vi "myRIO_BRig_FPGA_v3,41.vi"() -> ()   [LabVIEW 2014]
uses:
  <vilib>/rvi/FXPMathLib/FxpDiv/subVIs/nifxpmath_Div_SimConfig.ctl
  <vilib>/rvi/FXPMathLib/FxpSinAndCos/subVIs/nifxpmath_SinAndCos_SimConfig.ctl
  <vilib>/rvi/FXPMathLib/FxpDiv/simVIs/DllFxpDivTemp_sub.vi
  <vilib>/rvi/FXPMathLib/FxpSinAndCos/simVIs/DllFxpSinAndCosTemp_sub.vi
  <vilib>/rvi/Emulation/niFpgaGetClockAttributes.vi
  <vilib>/rvi/Emulation/niFpgaSctlEmulationGetInTimedLoop.vi
  <vilib>/rvi/Emulation/niFpgaEmulationReportErrorSimple.vi
  <vilib>/rvi/eio/common/nirviEmuTemplateMethod_errors.vi
  <vilib>/rvi/Emulation/niFpgaCriticalErrorInLSC.vi
  <vilib>/rvi/FXPMathLib/FxpDiv/XNode/nifxpmath_Div.xnode
  <vilib>/rvi/FXPMathLib/FxpMul/XNode/nifxpmath_Multiplier.xnode
  <vilib>/rvi/FXPMathLib/FxpSinAndCos/XNode/nifxpmath_SinAndCos.xnode
  <vilib>/rvi/FXPMathLib/FxpSub/XNode/nifxpmath_Sub.xnode
  <vilib>/eio/EIONode/EIONode.xnode
  <vilib>/rvi/FXPMathLib/sim/FxpSim.dll
panel:
  in  "laser_Nshutter":u32=100
  in  "AnaOut_0":u16
  in  "laser_Nvalley":u32=100
  in  "laser_Npeak":u32=100
  in  "laserledMTrig":bool
  in  "laser_selWro_Ntotal":u32=100
  in  "laser_selWro_NDelay":u32
  in  "laser_selRew_Ntotal":u32=100
  in  "laser_selRew_Ndelay":u32
  in  "laserResponse_reward_LED":bool
  in  "laserResponse_wrong_LED":bool
  out "SelectWrong":bool
  out "SelectReward":bool
  in  "laserResponse_wrong":bool
  in  "laserResponse_reward":bool
  in  "Left(F)_or_Right(T)":bool
  in  "ignoreWrong":bool
  in  "SelectionState":bool
  in  "laserMTrig":bool
  in  "FPGA_Stop":bool
  in  "audioTrigger_L":bool
  in  "audioTrigger_R":bool
  in  "audioFreq_L_Hz":u16=1000 min=1000 max=14000 step=1000
  in  "audioAmp_L":u16=1 min=1 max=32767 step=1
  in  "audioFreq_R_Hz":u16=1000 min=1000 max=14000 step=1000
  in  "audioAmp_R":u16=1 min=1 max=32767 step=1
  in  "A3_SL":bool
  in  "A1_SR":bool
  in  "Counts_Reset":bool
  out "A4_LickR":u32
  out "A2_LickL":u32
  in  "A6_Act":bool
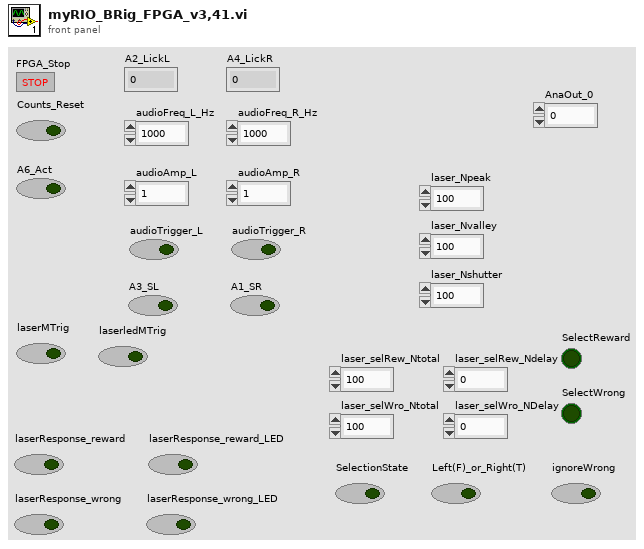
[diagram p1: front panel]
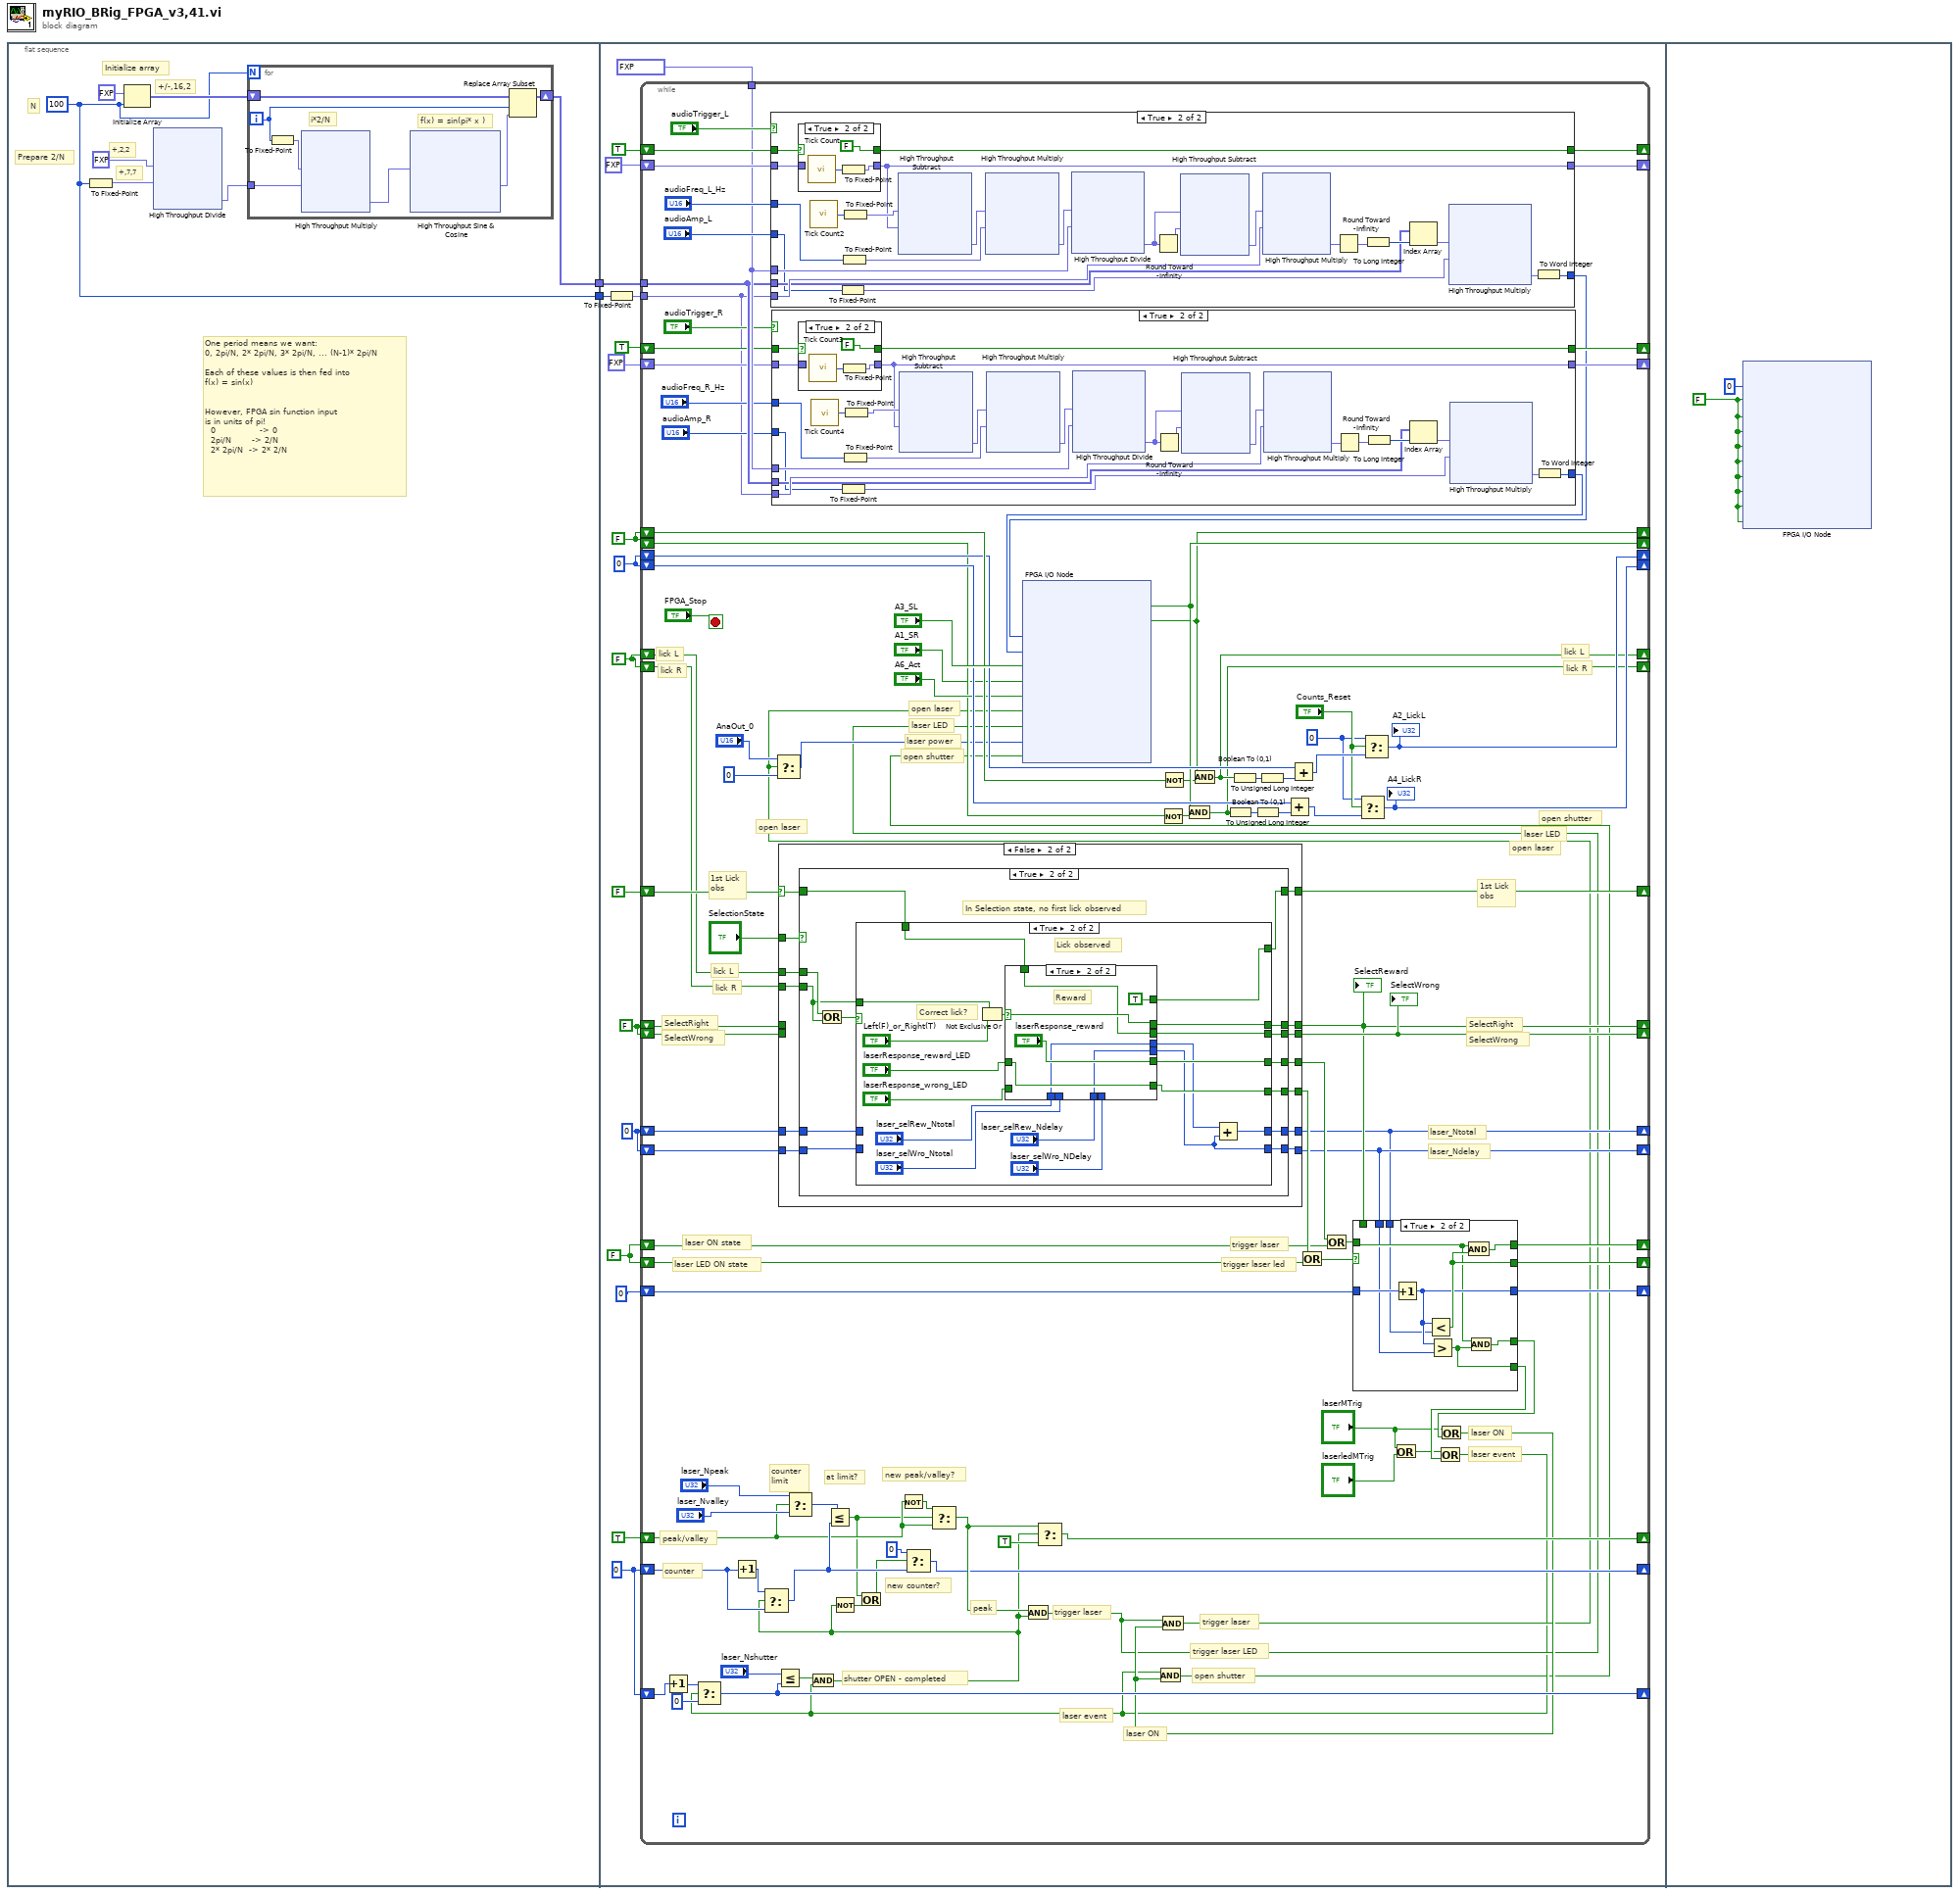
[diagram p0: block diagram]
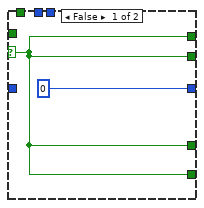
[diagram p2: hidden frame]
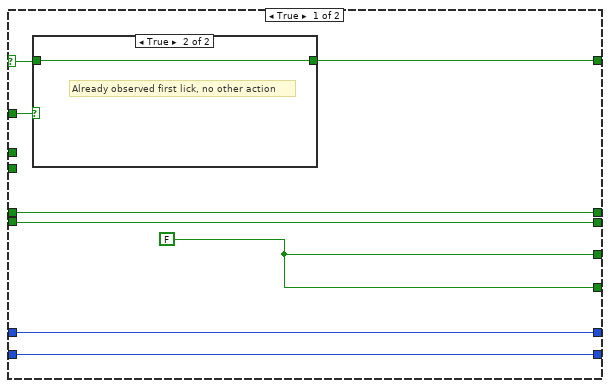
[diagram p3: hidden frame]
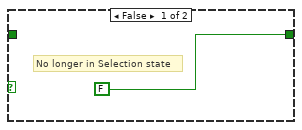
[diagram p4: hidden frame]
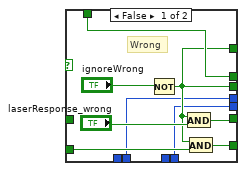
[diagram p7: hidden frame]
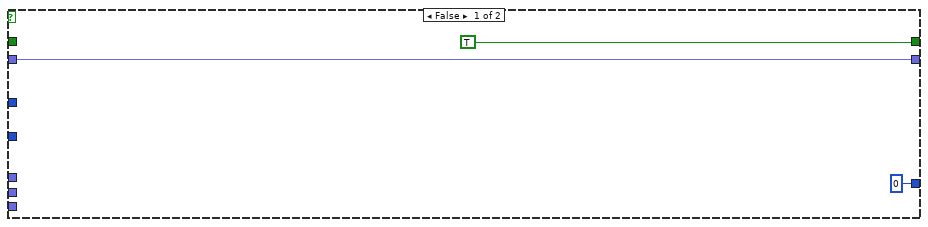
[diagram p8: hidden frame]
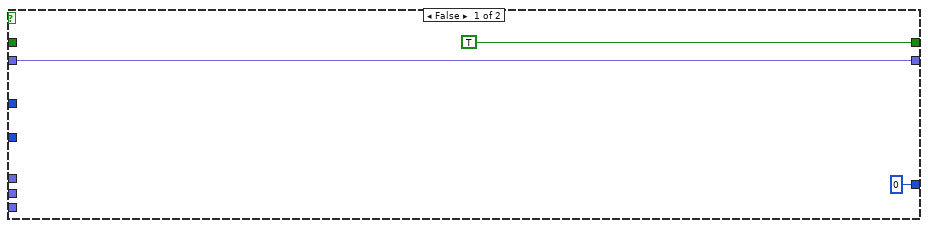
[diagram p10: hidden frame]
diagram:
  n1 = flat-sequence {
    tunnel: [w4] -> w2
    tunnel: [w3] -> w1
    tunnel: w2 -> [w86]
    tunnel: w1 -> [w88]
    frame #0 {
      w3 = 100 ("dimension size")
      # "N"
      # "+,7,7"
      # "+,2,2"
      # "+/-,16,2"
      # "Prepare 2/N"
      # "One period means we want:\n0, 2pi/N, 2* 2pi/N, 3* 2pi/N, ... (N-1)* 2pi/N\n\nEach of these values is then fed into\nf(x) = sin(x)\n\n\nHowever, FPGA sin function input\nis in units of pi!\n  0               -> 0\n  2pi/N       -> 2/N\n  2* 2pi/N  -> 2* 2/N"
      # "Initialize array"
      n2 = To Fixed-Point(number=w3) -> (fixed-point=w6:fxp<+,7,7>)  [unwired: 1 in]
      n3 = Initialize Array(fxp<+/-,16,2> 0.0 ("element"), w3) -> (w9:fxp<+/-,16,2>[])
      n4 = xnode "High Throughput Divide"("x"=fxp<+,2,2> 2.0, "y"=w6) -> ("x/y"=w5:fxp<+,27,0>)
      n5 = for {
        N: w3 -> [_]
        shift-right: [w42] -> w4
        shift-left: w9 -> [w43]
        tunnel: w5 -> [w38]
        i -> [w41]
        # "f(x) = sin(pi* x )"
        # "i*2/N"
        n6 = To Fixed-Point(number=w41) -> (fixed-point=w39:fxp<+,7,7>)  [unwired: 1 in]
        n7 = xnode ("High Throughput Multiply")("x"=w39, "y"=w38) -> ("x*y"=w37:fxp<+,34,7>)
        n8 = xnode "High Throughput Sine & Cosine"("x (pi)"=w37) -> ("sin(x)"=w40:fxp<+/-,16,2>)  [unwired: 1 out]
        n9 = Replace Array Subset(array=w43, new element=w40, index=w41) -> (w42:fxp<+/-,16,2>[])
      }
    }
    frame #1 {
      w74 = u32 0
      w76 = u32 0
      w78 = FALSE
      w77 = FALSE
      w81 = FALSE
      w82 = FALSE
      w83 = u32 0
      n10 = To Fixed-Point(number=w88) -> (fixed-point=w87:fxp<+,7,7>)  [unwired: 1 in]
      n11 = while {
        shift-right: [w187] -> _
        shift-left: TRUE -> [w191]
        shift-right: [w186] -> _
        shift-left: fxp<+,32,32> 0.0 -> [w190]
        tunnel: fxp<+,17,26> 40000000.0 -> [w185]
        tunnel: w87 -> [w178]
        tunnel: w86 -> [w184]
        shift-right: [w177] -> _
        shift-left: TRUE -> [w183]
        shift-right: [w176] -> _
        shift-left: fxp<+,32,32> 0.0 -> [w182]
        shift-right: [w154] -> _
        shift-left: w83 -> [w166]
        shift-right: [w157] -> _
        shift-left: w83 -> [w170]
        shift-right: [w158] -> _
        shift-left: w82 -> [w161]
        shift-right: [w155] -> _
        shift-left: w82 -> [w167]
        shift-right: [w152] -> _
        shift-left: FALSE -> [w151]
        shift-right: [w150] -> _
        shift-left: w81 -> [w148]
        shift-right: [w149] -> _
        shift-left: w81 -> [w147]
        shift-right: [w137] -> _
        shift-left: w77 -> [w139]
        shift-right: [w145] -> _
        shift-left: u32 0 -> [w146]
        shift-right: [w131] -> _
        shift-left: w78 -> [w143]
        shift-right: [w144] -> _
        shift-left: w78 -> [w142]
        shift-right: [w138] -> _
        shift-left: w77 -> [w135]
        shift-right: [w127] -> _
        shift-left: w76 -> [w130]
        shift-right: [w128] -> _
        shift-left: w76 -> [w129]
        shift-right: [w111] -> _
        shift-left: w74 -> [w121]
        shift-right: [w112] -> _
        shift-left: TRUE -> [w115]
        shift-right: [w100] -> _
        shift-left: w74 -> [w104]
        stop <- "FPGA_Stop" stop-if-true
        w163 = u32 0
        # "open shutter"
        # "laser LED"
        # "open laser"
        # "open laser"
        # "trigger laser LED"
        # "trigger laser"
        # "open shutter"
        # "laser ON"
        # "laser power"
        # "open laser"
        # "laser LED"
        # "open shutter"
        # "shutter OPEN - completed"
        # "trigger laser"
        # "peak"
        # "laser event"
        # "new peak/valley?"
        # "counter"
        # "peak/valley"
        # "new counter?"
        # "at limit?"
        # "counter\nlimit"
        # "laser_Ndelay"
        # "laser_Ntotal"
        # "laser event"
        # "laser ON"
        # "laser LED ON state"
        # "laser ON state"
        # "SelectWrong"
        # "SelectRight"
        # "SelectWrong"
        # "SelectRight"
        # "lick R"
        # "lick L"
        # "1st Lick\nobs"
        # "1st Lick\nobs"
        # "lick R"
        # "lick L"
        # "lick R"
        # "lick L"
        # "trigger laser led"
        # "trigger laser"
        n12 = Increment(x=w104) -> (x+1=w103:u32)
        n13 = Increment(x=w121) -> (x+1=w120:u32)
        n14 = case shown="True" "audioTrigger_L" {
          tunnel: w191 -> [_ w366]
          tunnel: w190 -> [w342 w365]
          tunnel: "audioFreq_L_Hz" -> [_ w362]
          tunnel: w185 -> [_ w359]
          tunnel: [w342 w343] -> w186
          tunnel: [TRUE w356] -> w187
          tunnel: w178 -> [_ w355]
          tunnel: w184 -> [_ w350]
          tunnel: "audioAmp_L" -> [_ w348]
          tunnel: [i16 0 w345] -> w173
          frame False {
          }
          frame True {
            n15 = case shown="True" w366 {
              selector: w366 -> [w395 _]
              tunnel: [w395 FALSE] -> w356
              tunnel: w365 -> [w394 _]
              tunnel: [w394 w396] -> w343
              frame False {
              }
              frame True {
                n16 = call "Tick Count"() -> ("Tick Count(Ticks)"=w398:u32)
                n17 = To Fixed-Point(number=w398) -> (fixed-point=w396:fxp<+,32,32>)  [unwired: 1 in]
              }
            }
            n18 = call "Tick Count2"() -> ("Tick Count(Ticks)"=w364:u32)
            n19 = To Fixed-Point(number=w348) -> (fixed-point=w347:fxp<+,15,15>)  [unwired: 1 in]
            n20 = To Fixed-Point(number=w362) -> (fixed-point=w361:fxp<+,14,14>)  [unwired: 1 in]
            n21 = To Fixed-Point(number=w364) -> (fixed-point=w344:fxp<+,32,32>)  [unwired: 1 in]
            n22 = xnode "High Throughput Subtract"("x"=w344, "y"=w343) -> ("x-y"=w363:fxp<+,32,32>)
            n23 = xnode ("High Throughput Multiply")("x"=w363, "y"=w361) -> ("x*y"=w360:fxp<+,46,46>)
            n24 = xnode "High Throughput Divide"("x"=w360, "y"=w359) -> ("x/y"=w358:fxp<+,34,21>)
            n25 = Round Toward -Infinity(1:w358) -> (0:w357:fxp<+,21,21>)
            n26 = xnode "High Throughput Subtract"("x"=w358, "y"=w357) -> ("x-y"=w354:fxp<+,14,1>)
            n27 = xnode ("High Throughput Multiply")("x"=w354, "y"=w355) -> ("x*y"=w351:fxp<+,21,8>)
            n28 = Round Toward -Infinity(1:w351) -> (0:w353:fxp<+,8,8>)
            n29 = To Long Integer(number=w353) -> (32bit integer=w352:i32)
            n30 = Index Array(array=w350, index=w352) -> (element=w349:fxp<+/-,16,2>)
            n31 = xnode ("High Throughput Multiply")("x"=w349, "y"=w347) -> ("x*y"=w346:fxp<+/-,31,17>)
            n32 = To Word Integer(number=w346) -> (16bit integer=w345:i16)
          }
        }
        n33 = case shown="True" "audioTrigger_R" {
          tunnel: w183 -> [_ w307]
          tunnel: w182 -> [w283 w306]
          tunnel: "audioFreq_R_Hz" -> [_ w303]
          tunnel: w185 -> [_ w300]
          tunnel: [w283 w284] -> w176
          tunnel: [TRUE w297] -> w177
          tunnel: w178 -> [_ w296]
          tunnel: w184 -> [_ w291]
          tunnel: "audioAmp_R" -> [_ w289]
          tunnel: [i16 0 w286] -> w174
          frame False {
          }
          frame True {
            n34 = case shown="True" w307 {
              selector: w307 -> [w336 _]
              tunnel: [w336 FALSE] -> w297
              tunnel: w306 -> [w335 _]
              tunnel: [w335 w337] -> w284
              frame False {
              }
              frame True {
                n35 = call "Tick Count3"() -> ("Tick Count(Ticks)"=w339:u32)
                n36 = To Fixed-Point(number=w339) -> (fixed-point=w337:fxp<+,32,32>)  [unwired: 1 in]
              }
            }
            n37 = call "Tick Count4"() -> ("Tick Count(Ticks)"=w305:u32)
            n38 = To Fixed-Point(number=w289) -> (fixed-point=w288:fxp<+,15,15>)  [unwired: 1 in]
            n39 = To Fixed-Point(number=w303) -> (fixed-point=w302:fxp<+,14,14>)  [unwired: 1 in]
            n40 = To Fixed-Point(number=w305) -> (fixed-point=w285:fxp<+,32,32>)  [unwired: 1 in]
            n41 = xnode "High Throughput Subtract"("x"=w285, "y"=w284) -> ("x-y"=w304:fxp<+,32,32>)
            n42 = xnode ("High Throughput Multiply")("x"=w304, "y"=w302) -> ("x*y"=w301:fxp<+,46,46>)
            n43 = xnode "High Throughput Divide"("x"=w301, "y"=w300) -> ("x/y"=w299:fxp<+,34,21>)
            n44 = Round Toward -Infinity(1:w299) -> (0:w298:fxp<+,21,21>)
            n45 = xnode "High Throughput Subtract"("x"=w299, "y"=w298) -> ("x-y"=w295:fxp<+,14,1>)
            n46 = xnode ("High Throughput Multiply")("x"=w295, "y"=w296) -> ("x*y"=w292:fxp<+,21,8>)
            n47 = Round Toward -Infinity(1:w292) -> (0:w294:fxp<+,8,8>)
            n48 = To Long Integer(number=w294) -> (32bit integer=w293:i32)
            n49 = Index Array(array=w291, index=w293) -> (element=w290:fxp<+/-,16,2>)
            n50 = xnode ("High Throughput Multiply")("x"=w290, "y"=w288) -> ("x*y"=w287:fxp<+/-,31,17>)
            n51 = To Word Integer(number=w287) -> (16bit integer=w286:i16)
          }
        }
        n52 = case shown="False" w151 {
          selector: w151 -> [w210 w225]
          tunnel: "SelectionState" -> [w212 w227]
          tunnel: [w211 w226] -> w152
          tunnel: w148 -> [_ w224]
          tunnel: w147 -> [_ w223]
          tunnel: [w209 w222] -> w136
          tunnel: [w207 w221] -> w131
          tunnel: [w208 w220] -> w144
          tunnel: w143 -> [w207 _]
          tunnel: w142 -> [w208 _]
          tunnel: [w209 w219] -> w140
          tunnel: [w206 w218] -> w127
          tunnel: [w205 w217] -> w128
          tunnel: w130 -> [w206 w216]
          tunnel: w129 -> [w205 w215]
          frame True {
            w209 = FALSE
            n53 = case shown="True" w212 {
              tunnel: [FALSE w214] -> w211
              tunnel: w210 -> [_ w214]
              frame False {
                # "No longer in Selection state"
              }
              frame True {
                # "Already observed first lick, no other action"
              }
            }
          }
          frame False {
            n54 = case shown="True" w227 {
              tunnel: [w230 w240] -> w226
              tunnel: w225 -> [w230 w236]
              tunnel: w224 -> [_ w242]
              tunnel: w223 -> [_ w241]
              tunnel: [w230 w239] -> w222
              tunnel: [w230 w238] -> w221
              tunnel: [w230 w237] -> w220
              tunnel: [w230 w235] -> w219
              tunnel: [w229 w234] -> w218
              tunnel: [w228 w233] -> w217
              tunnel: w216 -> [w229 w232]
              tunnel: w215 -> [w228 w231]
              frame False {
                # "Not in Selection state"
              }
              frame True {
                # "In Selection state, no first lick observed"
                n55 = Or(x=w242, y=w241) -> (x .or. y?=w243:bool)
                n56 = case shown="True" w243 {
                  tunnel: w241 -> [_ w263]
                  tunnel: [w246 w256] -> w240
                  tunnel: [w246 w261] -> w239
                  tunnel: [w246 w260] -> w238
                  tunnel: [w246 w259] -> w237
                  tunnel: w236 -> [w246 w258]
                  tunnel: [w246 w257] -> w235
                  tunnel: [w245 w249] -> w234
                  tunnel: [w244 w247] -> w233
                  tunnel: w232 -> [w245 _]
                  tunnel: w231 -> [w244 _]
                  frame False {
                  }
                  frame True {
                    # "Correct lick?"
                    # "Lick observed"
                    n57 = Not Exclusive Or(1:"Left(F)_or_Right(T)", 2:w263) -> (0:w262:bool)
                    n58 = case shown="True" w262 {
                      selector: w262 -> [_ w279]
                      tunnel: [w270 "laserResponse_reward"] -> w261
                      tunnel: [w268 w275] -> w259
                      tunnel: [w272 w279] -> w260
                      tunnel: w258 -> [w272 w275]
                      tunnel: [w269 w277] -> w257
                      tunnel: [w268 TRUE] -> w256
                      tunnel: "laserResponse_reward_LED" -> [_ w277]
                      tunnel: "laserResponse_wrong_LED" -> [w267 _]
                      tunnel: "laser_selRew_Ntotal" -> [_ w274]
                      tunnel: "laser_selWro_Ntotal" -> [w265 _]
                      tunnel: "laser_selRew_Ndelay" -> [_ w276]
                      tunnel: "laser_selWro_NDelay" -> [w266 _]
                      tunnel: [w266 w276] -> w247
                      tunnel: [w265 w274] -> w248
                      frame False {
                        # "Wrong"
                        n59 = Not(x="ignoreWrong") -> (.not. x?=w268:bool)
                        n60 = And(x=w268, y="laserResponse_wrong") -> (x .and. y?=w270:bool)
                        n61 = And(x=w268, y=w267) -> (x .and. y?=w269:bool)
                      }
                      frame True {
                        # "Reward"
                      }
                    }
                    n62 = Add(x=w248, y=w247) -> (x+y=w249:u32)
                  }
                }
              }
            }
          }
        }
        "SelectWrong" <- w144
        "SelectReward" <- w131
        n63 = Select(t="laser_Npeak", s=w115, f="laser_Nvalley") -> (s? t:f=w123:u32)
        n64 = Not(x=w115) -> (.not. x?=w116:bool)
        n65 = Not(x=w161) -> (.not. x?=w160:bool)
        n66 = Not(x=w167) -> (.not. x?=w156:bool)
        n67 = Or(x=w140, y=w139) -> (x .or. y?=w141:bool)
        n68 = Or(x=w136, y=w135) -> (x .or. y?=w134:bool)
        n69 = case shown="True" w141 {
          selector: w141 -> [w194 _]
          tunnel: w146 -> [_ w204]
          tunnel: [u32 0 w201] -> w145
          tunnel: [w194 w202] -> w137
          tunnel: [w194 w203] -> w138
          tunnel: w134 -> [_ w200]
          tunnel: [w194 w199] -> w132
          tunnel: [w194 w198] -> w133
          tunnel: w131 -> [_ _]
          tunnel: w128 -> [_ w197]
          tunnel: w127 -> [_ w196]
          frame False {
          }
          frame True {
            n70 = Increment(x=w204) -> (x+1=w201:u32)
            n71 = Less?(x=w201, y=w196) -> (x < y?=w202:bool)
            n72 = Greater?(x=w201, y=w197) -> (0:w199:bool)
            n73 = And(x=w200, y=w202) -> (x .and. y?=w203:bool)
            n74 = And(x=w200, y=w199) -> (x .and. y?=w198:bool)
          }
        }
        n75 = Or(x="laserMTrig", y="laserledMTrig") -> (x .or. y?=w125:bool)
        n76 = Or(x=w125, y=w132) -> (x .or. y?=w93:bool)
        n77 = Select(t=w103, s=w93, f=u32 0) -> (s? t:f=w100:u32)
        n78 = Less Or Equal?(x="laser_Nshutter", y=w100) -> (x <= y?=w99:bool)
        n79 = And(x=w99, y=w93) -> (x .and. y?=w97:bool)
        n80 = Select(t=w120, s=w97, f=w121) -> (s? t:f=w119:u32)
        n81 = Less Or Equal?(x=w123, y=w119) -> (x <= y?=w109:bool)
        n82 = Not(x=w97) -> (.not. x?=w110:bool)
        n83 = Or(x=w109, y=w110) -> (x .or. y?=w108:bool)
        n84 = Select(t=u32 0, s=w108, f=w119) -> (s? t:f=w111:u32)
        n85 = Select(t=w116, s=w109, f=w115) -> (s? t:f=w114:bool)
        n86 = And(x=w114, y=w97) -> (x .and. y?=w94:bool)
        n87 = Select(t=w114, s=w97, f=TRUE) -> (s? t:f=w112:bool)
        n88 = Or(x="laserMTrig", y=w133) -> (x .or. y?=w96:bool)
        n89 = And(x=w93, y=w96) -> (x .and. y?=w92:bool)
        n90 = And(x=w94, y=w96) -> (x .and. y?=w95:bool)
        n91 = Select(t="AnaOut_0", s=w95, f=u16 0) -> (s? t:f=w107:u16)
        n92 = xnode "FPGA I/O Node"("AudioOut/Left"=w173, "AudioOut/Right"=w174, "ConnectorA/DIO3"="A3_SL", "ConnectorA/DIO1"="A1_SR", "ConnectorA/DIO7"="A6_Act", "ConnectorA/DIO0"=w95, "ConnectorA/DIO14"=w94, "ConnectorB/AO0"=w107, "ConnectorA/DIO6"=w92) -> ("ConnectorA/DIO4"=w158:bool, "ConnectorA/DIO2"=w155:bool)  [unwired: 11 in, 11 out]
        n93 = And(x=w158, y=w160) -> (x .and. y?=w149:bool)
        n94 = And(x=w155, y=w156) -> (x .and. y?=w150:bool)
        n95 = Boolean To (0,1)(Boolean=w149) -> (0, 1=w172:i16)
        n96 = Boolean To (0,1)(Boolean=w150) -> (0, 1=w169:i16)
        n97 = To Unsigned Long Integer(number=w172) -> (unsigned 32bit integer=w171:u32)
        n98 = To Unsigned Long Integer(number=w169) -> (unsigned 32bit integer=w168:u32)
        n99 = Add(x=w170, y=w171) -> (x+y=w159:u32)
        n100 = Add(x=w166, y=w168) -> (x+y=w165:u32)
        n101 = Select(t=w163, s="Counts_Reset", f=w159) -> (s? t:f=w157:u32)
        "A4_LickR" <- w157
        n102 = Select(t=w163, s="Counts_Reset", f=w165) -> (s? t:f=w154:u32)
        "A2_LickL" <- w154
      }
    }
    frame #2 {
      w399 = FALSE ("ConnectorA/DIO3")
      n103 = xnode "FPGA I/O Node"("ConnectorB/AO0"=u16 0 ("ConnectorA/AO0"), "ConnectorA/DIO0"=w399, "ConnectorA/DIO1"=w399, "ConnectorA/DIO2"=w399, "ConnectorA/DIO3"=w399, "ConnectorA/DIO4"=w399, "ConnectorA/DIO5"=w399, "ConnectorA/DIO6"=w399, "ConnectorA/DIO7"=w399, "ConnectorA/DIO14"=w399) -> ()  [unwired: 10 in, 10 out]
    }
  }
